vi "TCP - Write and Read a Synchronous Message.vi"(8 "error in":errorcluster, 10 "Message to Send":string, 11 "TCP Network Connection in":refnum<k5>) -> (0 "error out":errorcluster, 2 "Received Text":string, 3 "TCP Network Connection out":refnum<k5>)   [LabVIEW 2021]
doc: "Send a TCP message and listen for the response. \nThe linefeed character is used to detect the end of the response message."
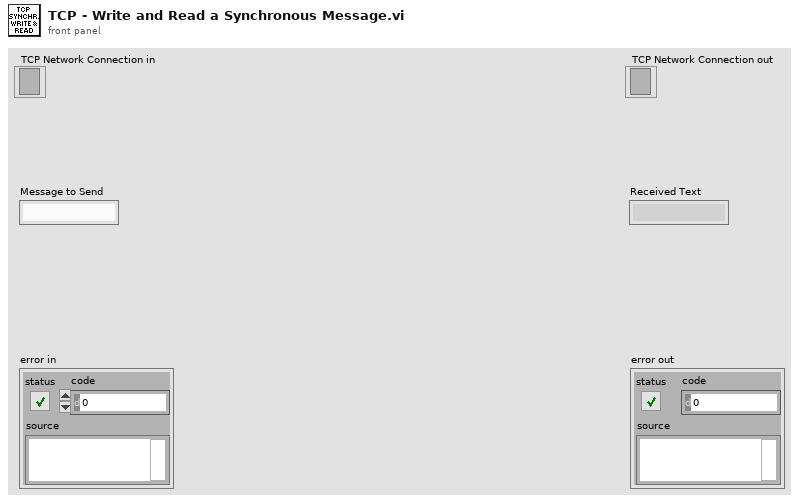
[diagram p1: front panel]
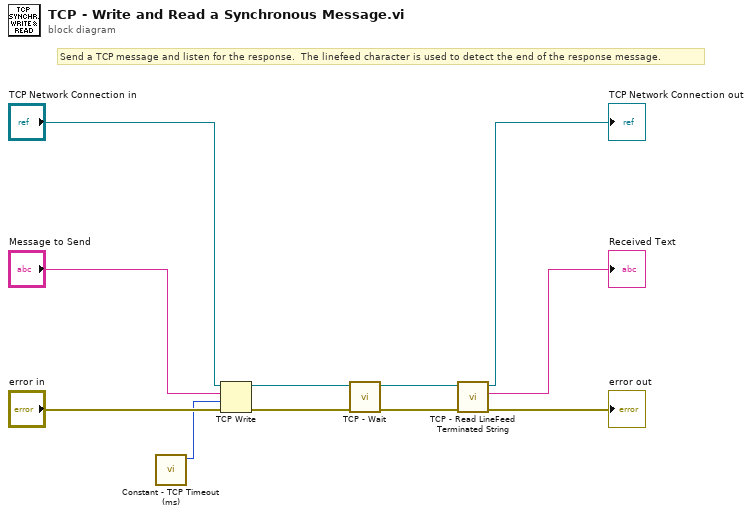
[diagram p0: block diagram]
diagram:
  # "Send a TCP message and listen for the response.  The linefeed character is used to detect the end of the response message."
  n1 = call "Constant - TCP Timeout (ms).vi"() -> ("timeout (ms)"=w1:i32)  [unwired: 11 in]
  n2 = TCP Write(connection ID="TCP Network Connection in", data in="Message to Send", error in (no error)="error in", 9:w1) -> (connection ID out=w5:refnum<k5>, error out=w10:errorcluster)  [unwired: 1 out]
  n3 = call "TCP - Wait.vi"("error in"=w10, "TCP Network Connection in"=w5) -> ("error out"=w9:errorcluster, "TCP Network Connection out"=w4:refnum<k5>)  [unwired: 8 in]
  n4 = call "TCP - Read LineFeed Terminated String.vi"("error in"=w9, "TCP Network Connection in"=w4) -> ("error out"=→"error out":errorcluster, "Received Text"=→"Received Text":string, "TCP Network Connection out"=→"TCP Network Connection out":refnum<k5>)  [unwired: 7 in]
